vi "getNyanNext.vi"(1 "getNya?":bool) -> (0 "Nya":picture)   [LabVIEW 2014]
uses:
  <vilib>/Utility/sysdir.llb/System Directory Type.ctl
  <vilib>/Utility/miscctls.llb/LVBoundsTypeDef.ctl
panel:
  out "reGetNya":bool
  out "fileNumber":i64
  out "numberOfTheNyas":i64
  in  "don'tWantNoMoreNya?":bool
  in  "saveNya?":bool
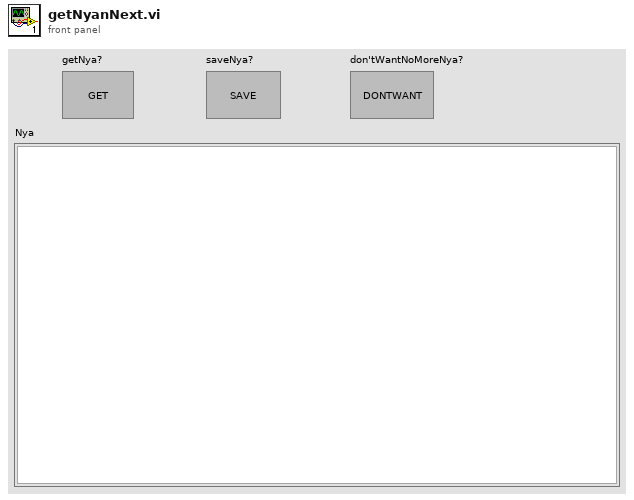
[diagram p1: front panel]
types:
  T1 = enum16{"Native", "Native Command Line", "UNIX", "Macintosh", "DOS"}
  T2 = typedef "LVBoundsTypeDef.ctl" = cluster{"Width":u32, "Height":u32}
  T3 = typedef "System Directory Type.ctl" = i32
  T4 = typedef "imagedata.ctl" = cluster{"image type":i32, "image depth":i32, "image":u8[], "mask":u8[], "colors":u32[], "Rectangle":cluster{"left":i16, "top":i16, "right":i16, "bottom":i16}}
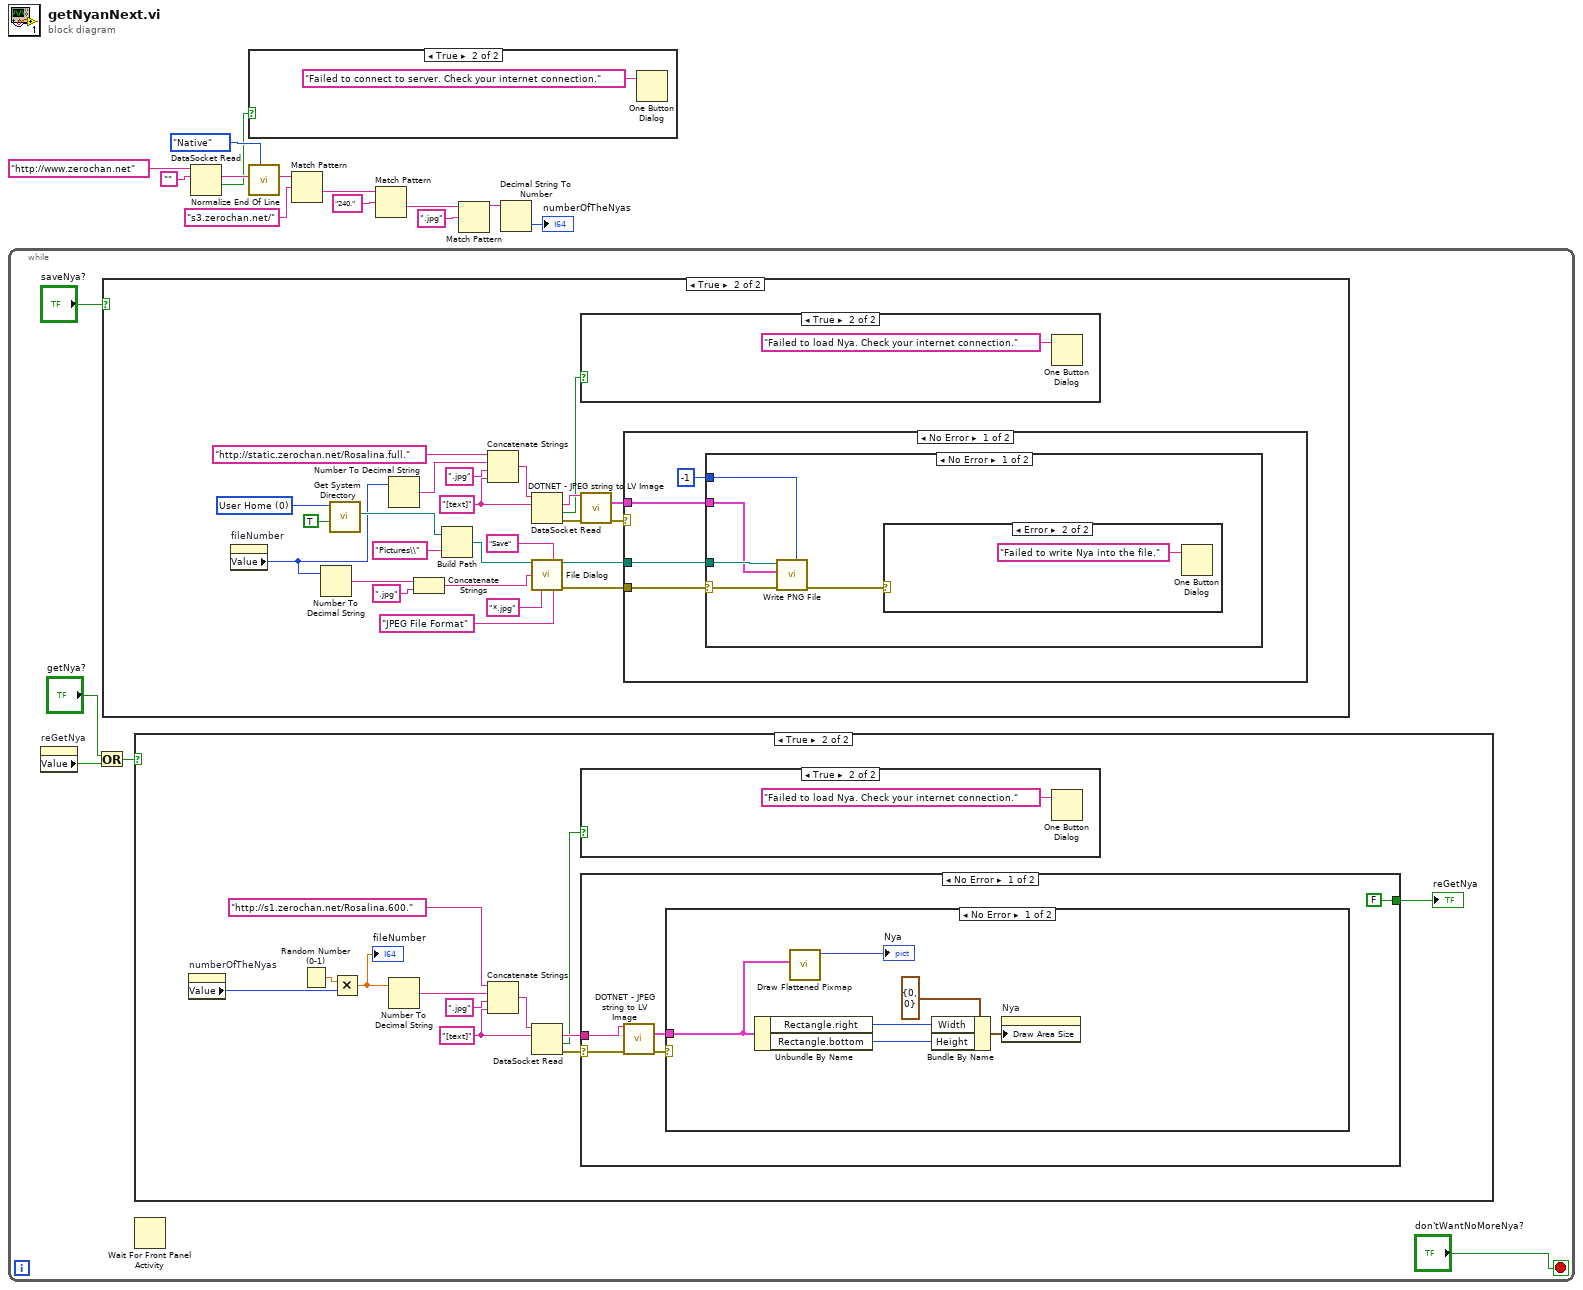
[diagram p0: block diagram]
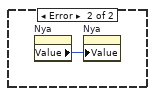
[diagram p6: hidden frame]
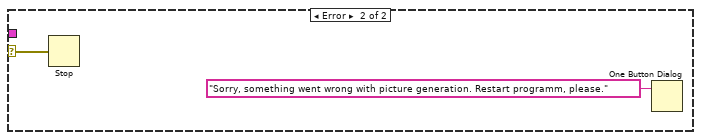
[diagram p10: hidden frame]
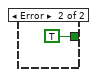
[diagram p11: hidden frame]
diagram:
  n1 = while {
    stop <- "don'tWantNoMoreNya?" stop-if-true
    n2 = property on="reGetNya" class="Bool (strict)"() -> ("Value"=w14:bool)  [unwired: 2 in, 2 out]
    n3 = Or(x="getNya?", y=w14) -> (x .or. y?=w15:bool)
    n4 = case shown="True" "saveNya?" {
      frame False {
      }
      frame True {
        w33 = T3 0 items=["User Home"=0, "User Desktop"=1, "User Documents"=2, "User Application Data"=3, "User Preferences"=4, "User Temporary"=5, "Public Documents"=6, "Public Application Data"=7, "Public Preferences"=8, "Public Cache"=13, "System Core Libraries"=9, "System Installed Libraries"=10, "Application Files"=11, "Boot Volume Root"=12] ("system directory type")
        w37 = "[text]"
        n5 = property on="fileNumber" class="DigNum (strict)"() -> ("Value"=w20:i64)  [unwired: 2 in, 2 out]
        n6 = Number To Decimal String(number=w20) -> (decimal integer string=w42:string)  [unwired: 1 in]
        n7 = call <vilib>:"Get System Directory.vi"("create directory if not found? (F)"=TRUE, "system directory type"=w33) -> ("system directory"=w32:path)  [unwired: 9 in]
        n8 = Number To Decimal String(number=w20) -> (decimal integer string=w39:string)  [unwired: 1 in]
        n9 = Concatenate Strings(w42, ".jpg") -> (w41:string)
        n10 = Build Path(base path=w32, name or relative path="Pictures\\") -> (appended path=w30:path)
        n11 = Concatenate Strings("http://static.zerochan.net/Rosalina.full.", w39, ".jpg", w37) -> (w38:string)
        n12 = DataSocket Read(10:w37, 11:w38) -> (0:w35:errorcluster, 1:w19:bool, 2:w36:string)  [unwired: 3 in, 4 out]
        n13 = call "File Dialog"("start path"=w30, "button label"="Save", "default name"=w41, "pattern (all files)"="*.jpg", "pattern label"="JPEG File Format") -> ("selected path"=w23:path, "error out"=w24:errorcluster)  [unwired: 7 in, 2 out]
        n14 = case shown="True" w19 {
          frame False {
          }
          frame True {
            n15 = One Button Dialog(message="Failed to load Nya. Check your internet connection.") -> ()  [unwired: 1 in, 1 out]
          }
        }
        n16 = call "DOTNET - JPEG string to LV Image.vi"("JPEG String"=w36, "error in"=w35) -> ("LV Image"=w22:T4, "error out"=w21:errorcluster)  [unwired: 12 in]
        n17 = case shown="No Error" w21 {
          tunnel: w24 -> [w47 _]
          tunnel: w23 -> [w46 _]
          tunnel: w22 -> [w45 _]
          frame No Error {
            n18 = case shown="No Error" w47 {
              selector: w47 -> [w48 _]
              tunnel: w46 -> [w52 _]
              tunnel: w45 -> [w51 _]
              tunnel: -1 ("compression (default)") -> [w50 _]
              frame No Error {
                n19 = call <vilib>:"Write PNG File.vi"("compression (default)"=w50, "error in (no error)"=w48, "image data"=w51, "path to PNG file"=w52) -> ("error out"=w49:errorcluster)  [unwired: 6 in, 1 out]
                n20 = case shown="Error" w49 {
                  frame No Error {
                  }
                  frame Error {
                    n21 = One Button Dialog(message="Failed to write Nya into the file.") -> ()  [unwired: 1 in, 1 out]
                  }
                }
              }
              frame Error {
                n22 = property on="Nya" class="Pict"() -> ("Value"=w54:picture)  [unwired: 2 in, 2 out]
                n23 = property on="Nya" class="Pict"("Value"=w54) -> ()  [unwired: 2 in, 2 out]
              }
            }
          }
          frame Error {
          }
        }
      }
    }
    n24 = case shown="True" w15 {
      frame False {
      }
      frame True {
        w62 = "[text]"
        n25 = property on="numberOfTheNyas" class="DigNum (strict)"() -> ("Value"=w58:i64)  [unwired: 2 in, 2 out]
        n26 = Random Number (0-1)() -> (number: 0 to 1=w65:dbl)
        n27 = Multiply(x=w65, y=w58) -> (x*y=w57:dbl)
        "fileNumber" <- w57
        n28 = Number To Decimal String(number=w57) -> (decimal integer string=w64:string)  [unwired: 1 in]
        n29 = Concatenate Strings("http://s1.zerochan.net/Rosalina.600.", w64, ".jpg", w62) -> (w66:string)
        n30 = DataSocket Read(10:w62, 11:w66) -> (0:w59:errorcluster, 1:w56:bool, 2:w61:string)  [unwired: 3 in, 4 out]
        n31 = case shown="True" w56 {
          frame False {
          }
          frame True {
            n32 = One Button Dialog(message="Failed to load Nya. Check your internet connection.") -> ()  [unwired: 1 in, 1 out]
          }
        }
        n33 = case shown="No Error" w59 {
          selector: w59 -> [w71 _]
          tunnel: w61 -> [w72 _]
          tunnel: [FALSE TRUE] -> w55
          frame No Error {
            n34 = call "DOTNET - JPEG string to LV Image.vi"("JPEG String"=w72, "error in"=w71) -> ("LV Image"=w69:T4, "error out"=w70:errorcluster)  [unwired: 12 in]
            n35 = case shown="No Error" w70 {
              selector: w70 -> [_ w80]
              tunnel: w69 -> [w73 _]
              frame No Error {
                n36 = Unbundle By Name(w73) -> ("Rectangle.right"=w77:i16, "Rectangle.bottom"=w78:i16)
                n37 = call <vilib>:"Draw Flattened Pixmap.vi"("image data"=w73) -> ("new picture"=→"Nya":picture)  [unwired: 8 in]
                n38 = Bundle By Name(cluster=T2 {"Width"=0, "Height"=0} ("Draw Area Size"), "Width"=w77, "Height"=w78) -> (w76:T2)
                n39 = property on="Nya" class="Pict"("Draw Area Size"=w76) -> ()  [unwired: 2 in, 2 out]
              }
              frame Error {
                n40 = Stop(stop? (T)=w80) -> ()
                n41 = One Button Dialog(message="Sorry, something went wrong with picture generation. Restart programm, please.") -> ()  [unwired: 1 in, 1 out]
              }
            }
          }
          frame Error {
          }
        }
        "reGetNya" <- w55
      }
    }
    n42 = Wait For Front Panel Activity() -> ()  [unwired: 3 in, 1 out]
  }
  n43 = DataSocket Read(10:"", 11:"http://www.zerochan.net") -> (1:w1:bool, 2:w4:string)  [unwired: 3 in, 5 out]
  n44 = case shown="True" w1 {
    frame False {
    }
    frame True {
      n45 = One Button Dialog(message="Failed to connect to server. Check your internet connection.") -> ()  [unwired: 1 in, 1 out]
    }
  }
  n46 = call <vilib>:"Normalize End Of Line.vi"("end of line (Native)"=T1."Native", "string in"=w4) -> ("string out"=w3:string)  [unwired: 6 in]
  n47 = Match Pattern(string=w3, regular expression="s3.zerochan.net/") -> (after substring=w7:string)  [unwired: 1 in, 3 out]
  n48 = Match Pattern(string=w7, regular expression="240.") -> (after substring=w6:string)  [unwired: 1 in, 3 out]
  n49 = Match Pattern(string=w6, regular expression=".jpg") -> (before substring=w5:string)  [unwired: 1 in, 3 out]
  n50 = Decimal String To Number(string=w5) -> (number=→"numberOfTheNyas":i32)  [unwired: 2 in, 1 out]
